vi "fgt get sensor Unit.vi"(8 "error in (no error)":errorcluster, 11 "sensorIndex":u32) -> (0 "error out":errorcluster, 3 "unit out":T1)   [LabVIEW 2017, in "fgt_SDK.lvlib"]
doc: "Get current unit on selected sensor device, default value is \"µl/min\" for flowunits and 'mbar' for pressure sensors.\nEvery sensor read value and regulation command use this unit."
uses:
  fgt_SDK.lvlib
  TypeDefs/fgt_SENSOR_UNIT.ctl
  dlls/fgt_SDK_32.dll
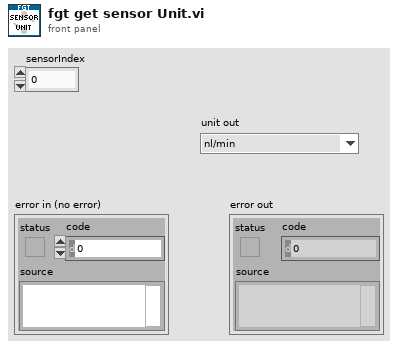
[diagram p1: front panel]
types:
  T1 = typedef "fgt_SDK.lvlib/fgt_SENSOR_UNIT.ctl" = enum16{"nl/min", "µl/s", "µl/min", "ul/h", "ml/min", "ml/h", "mbar", "PSI", "bar"}
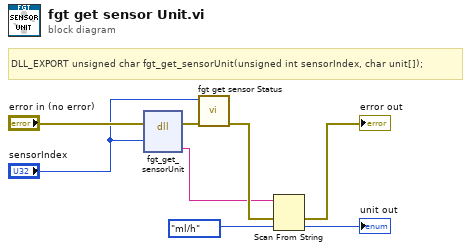
[diagram p0: block diagram]
diagram:
  # "DLL_EXPORT unsigned char fgt_get_sensorUnit(unsigned int sensorIndex, char unit[]);"
  n1 = dll-call lib="D:/Work/SDK git/fgt-sdk-labview/dlls/fgt_SDK_*.*" fn="fgt_get_sensorUnit"(error in="error in (no error)", "sensorIndex"="sensorIndex") -> (error out=w7:errorcluster, "unit"=w1:string)  [unwired: 5 in, 1 out]
  n2 = call "fgt get sensor Status.vi"("error in (no error)"=w7, "pressureIndex"="sensorIndex") -> ("error out"=w3:errorcluster)  [unwired: 9 in]
  n3 = Scan From String(input string=w1, error in=w3, default 1=fgt_SENSOR_UNIT."ml/h" ("unit out")) -> (error out=→"error out":errorcluster, output 1=→"unit out":T1)  [unwired: 2 in, 2 out]
